vi "LecturaCal.vi"(9 "T1":refnum<vi>) -> (0 "error out":errorcluster, 3 "Nom Sensor Temperatura":string)   [LabVIEW 2025]
uses:
  <vilib>/registry/registry.llb/Registry RtKey.ctl
  <vilib>/registry/registry.llb/Read Registry Value Simple STR.vi
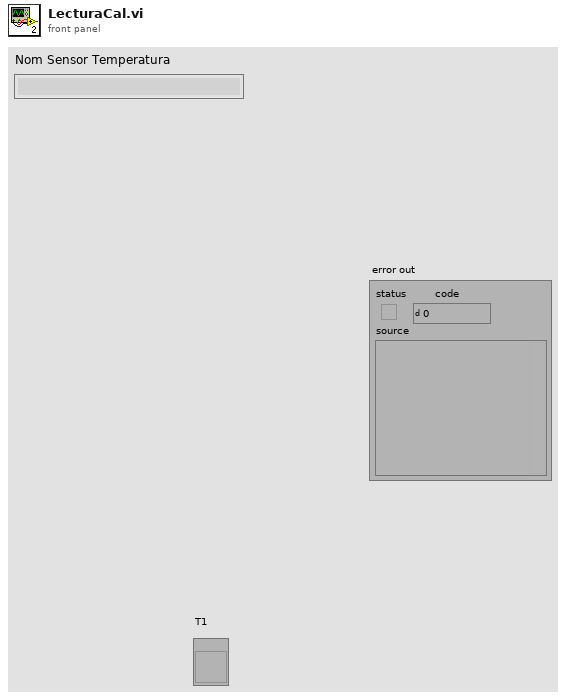
[diagram p1: front panel]
types:
  T1 = typedef "Registry RtKey.ctl" = enum32{"HKEY_CLASSES_ROOT", "HKEY_CURRENT_USER", "HKEY_LOCAL_MACHINE", "HKEY_USERS", "HKEY_PERFORMANCE_DATA", "HKEY_CURRENT_CONFIG", "HKEY_DYN_DATA"}
  T2 = typedef "Registry refnum.ctl" = refnum<k1>
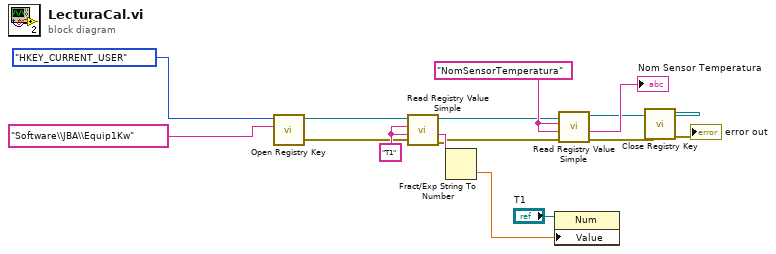
[diagram p0: block diagram]
diagram:
  w8 = "NomSensorTemperatura" ("value")
  w14 = "T1" ("value")
  n1 = call <vilib>:"Open Registry Key.vi"("subkey"="Software\\JBA\\Equip1Kw", "root key (HKEY_LOCAL_MACHINE)"=Registry_RtKey."HKEY_CURRENT_USER") -> ("error out"=w3:errorcluster, "refnum out"=w4:T2)  [unwired: 8 in]
  n2 = call-poly <vilib>:"Read Registry Value Simple.vi"("error in (no error)"=w3, "default data"=w14, "value"=w14, "refnum"=w4) -> ("error out"=w1:errorcluster, "String/Binary data"=w13:string, "refnum out"=w2:T2)  [unwired: 2 in, 1 out]
  n3 = Fract/Exp String To Number(string=w13) -> (number=w15:dbl)  [unwired: 3 in, 1 out]
  n4 = property on="Property Node" class="Num"(reference="T1", "Value"=w15) -> ()  [unwired: 1 in, 2 out]
  n5 = call-poly <vilib>:"Read Registry Value Simple.vi"("error in (no error)"=w1, "default data"=w8, "value"=w8, "refnum"=w2) -> ("error out"=w5:errorcluster, "String/Binary data"=→"Nom Sensor Temperatura":string, "refnum out"=w6:T2)  [unwired: 2 in, 1 out]
  n6 = call <vilib>:"Close Registry Key.vi"("error in (no error)"=w5, "refnum"=w6) -> ("error out"=→"error out":errorcluster)  [unwired: 5 in]
